vi "Read FDMR+data file.vi"(11 "Application Directory":path) -> (0 "Error Out":errorcluster, 1 "group names":string[](array[string]), 2 "Measurement parameters":T1={"F_start [GHz]"=380.0, "F_end [GHz]"=400.0, "Field [T]"=0.0, "Points [-]"=1, "Sampling Rate"=15, "ModA [G]"=1.0, "ModF [kHz]"=10.0, "Time const [ms]"=1.0, "Angle [°]"=-1.0, "Tmp [K]"=295.0, "Wait [min]"=0.0, "Repeat [-]"=0, "Comment"="", "Execute"=FALSE, "Auto-mod"=FALSE} {"Sampling Rate" items=["117 ks/S"=9, "58.6 kS/s"=10, "29.3 kS/s"=11, "14.6 kS/s"=12, "7.32 kS/s"=13, "3.66 kS/s"=14, "1.83 kS/s"=15]; "Time const [ms]" min=-1.0 max=330.0; "ModF [kHz]" min=0.2 max=120.0; "Repeat [-]" max=1048576; "Points [-]" max=50; "Wait [min]" max=1048576.0; "Field [T]" min=-16.0 max=16.0}, 3 "First acummulated spectrum":T3, 5 "TDMS File Path":path)   [LabVIEW 2022 SP3]
uses:
  Subsystem modules/Lock-in module/ctl/ADQ data.ctl
  Datatypes/FDMR+ script line.ctl
  Subsystem modules/Lock-in module/ctl/OSC sampling rate.ctl
  <vilib>/Utility/error.llb/Error Cluster From Error Code.vi
  <vilib>/ErrorRing/Error Ring.xnode
  Subsystem modules/Lock-in module/Lock-in module.lvlib
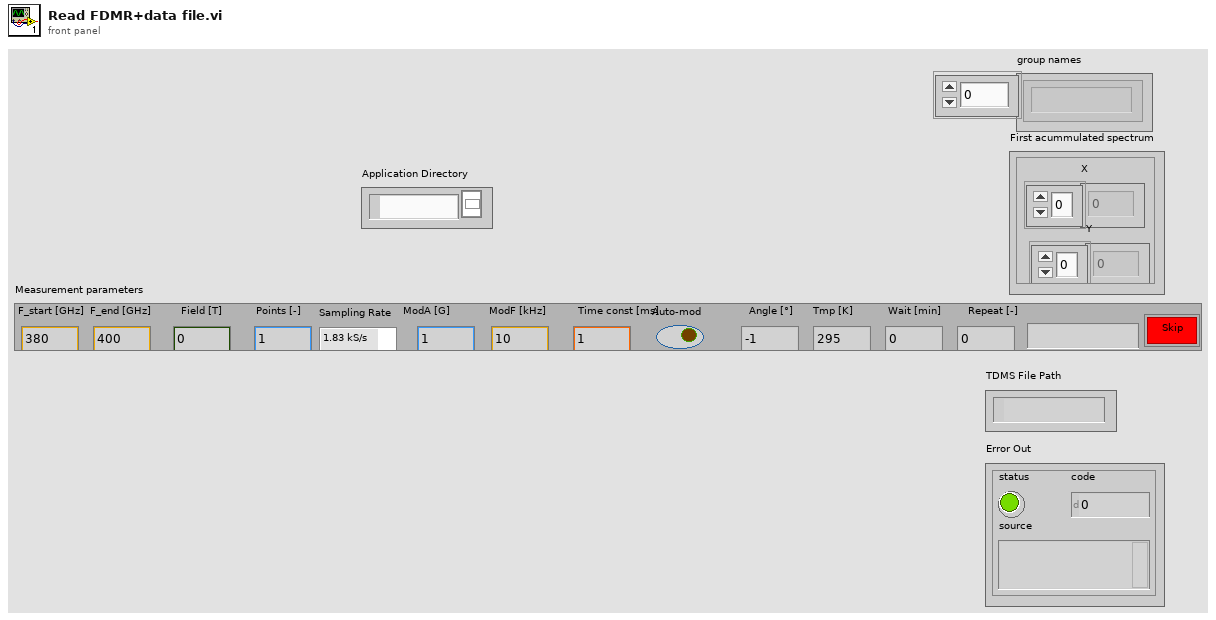
[diagram p1: front panel]
types:
  T1 = typedef "FDMR+ script line.ctl" = cluster{"F_start [GHz]":dbl, "F_end [GHz]":dbl, "Field [T]":dbl, "Points [-]":u32, "Sampling Rate":T2, "ModA [G]":dbl, "ModF [kHz]":dbl, "Time const [ms]":dbl, "Angle [°]":dbl, "Tmp [K]":dbl, "Wait [min]":dbl, "Repeat [-]":i32, "Comment":string, "Execute":bool, "Auto-mod":bool}
  T2 = typedef "OSC sampling rate.ctl" = u16
  T3 = typedef "Lock-in module.lvlib/ADQ data.ctl" = cluster{"X":sgl[], "Y":sgl[]}
  T4 = enum16{"open", "open or create", "create or replace", "create", "open (read-only)"}
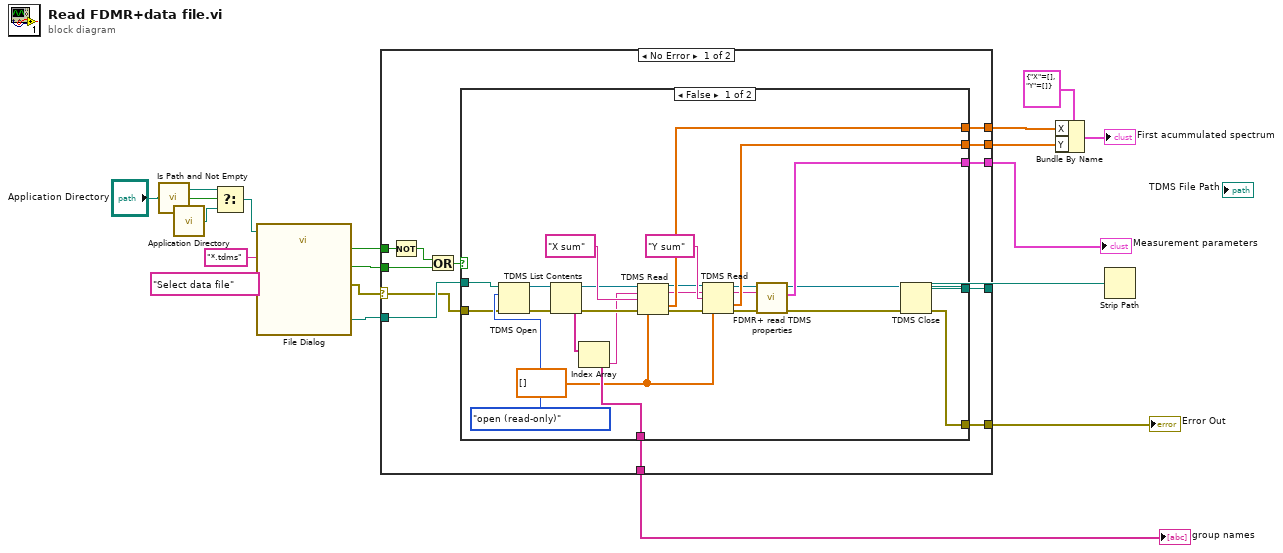
[diagram p0: block diagram]
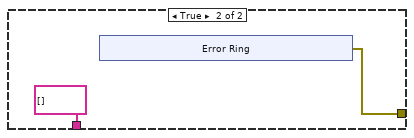
[diagram p2: hidden frame]
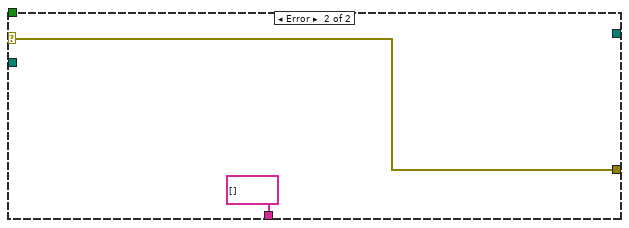
[diagram p3: hidden frame]
diagram:
  n1 = call <vilib>:"Is Path and Not Empty.vi"("path"="Application Directory") -> ("Is Path and Not Empty?"=w11:bool)  [unwired: 4 in]
  n2 = call <vilib>:"Application Directory.vi"() -> ("Application Directory"=w8:path)
  n3 = Select(t="Application Directory", s=w11, f=w8) -> (s? t:f=w9:path)
  n4 = call "File Dialog"("start path"=w9, "prompt"="Select data file", "pattern (all files)"="*.tdms") -> ("selected path"=w17:path, "exists"=w16:bool, "cancelled"=w15:bool, "error out"=w14:errorcluster)  [unwired: 9 in]
  n5 = case shown="No Error" w14 {
    selector: w14 -> [w23 w63]
    tunnel: w17 -> [w30 _]
    tunnel: w16 -> [w29 _]
    tunnel: w15 -> [w26 _]
    tunnel: [w25 _] -> w7
    tunnel: [w24 w63] -> w13
    tunnel: [w22 _] -> w3
    tunnel: [w21 string[] [] ("group names")] -> w4
    tunnel: [w20 _] -> w2
    tunnel: [w19 _] -> w1
    frame No Error {
      n6 = Not(x=w29) -> (.not. x?=w28:bool)
      n7 = Or(x=w28, y=w26) -> (x .or. y?=w27:bool)
      n8 = case shown="False" w27 {
        tunnel: w30 -> [w54 _]
        tunnel: [w55 _] -> w25
        tunnel: [w53 w57] -> w24
        tunnel: w23 -> [w51 _]
        tunnel: [w49 _] -> w22
        tunnel: [w43 string[] [] ("group names")] -> w21
        tunnel: [w41 _] -> w20
        tunnel: [w40 _] -> w19
        frame False {
          w39 = sgl[] []
          n9 = TDMS Open(8:w51, 10:T4."open (read-only)" ("operation (0:open)"), 11:w54) -> (0:w47:errorcluster, 3:w48:refnum<k34>)  [unwired: 4 in]
          n10 = TDMS List Contents(4:w47, 7:w48) -> (0:w45:errorcluster, 2:w43:string[], 3:w46:refnum<k34>)  [unwired: 1 in, 1 out]
          n11 = Index Array(array=w43) -> (element=w44:string)  [unwired: 1 in]
          n12 = TDMS Read(0:w46, 5:w44, 7:"X sum" ("channel name(s) in"), 11:w45, 12:w39) -> (4:w37:refnum<k34>, 6:w34:string, 10:w49:sgl[], 15:w38:errorcluster)  [unwired: 3 in, 2 out]
          n13 = TDMS Read(0:w37, 5:w34, 7:"Y sum" ("channel name(s) in"), 11:w38, 12:w39) -> (4:w35:refnum<k34>, 6:w33:string, 10:w40:sgl[], 15:w36:errorcluster)  [unwired: 3 in, 2 out]
          n14 = call "FDMR+ read TDMS properties.vi"("error in (no error)"=w36, "cahnnel group name in"=w33, "TDMS ref in"=w35) -> ("error out"=w31:errorcluster, "FDMR+ measurement parameters"=w41:T1, "TDMS ref out"=w32:refnum<k34>)  [unwired: 5 in, 1 out]
          n15 = TDMS Close(8:w31, 11:w32) -> (0:w53:errorcluster, 3:w55:path)
        }
        frame True {
          n16 = xnode "Error Ring"() -> ("error out"=w57:errorcluster)
        }
      }
    }
    frame Error {
    }
  }
  "Error Out" <- w13
  "group names" <- w4
  "Measurement parameters" <- w2
  n17 = Bundle By Name(cluster=T3 {"X"=[], "Y"=[]} ("ADQ data"), "X"=w3, "Y"=w1) -> (→"First acummulated spectrum":T3)
  n18 = Strip Path(path=w7) -> ()  [unwired: 2 out]
